vi "createChannel.vi"(8 "error in (no error)":errorcluster, 11 "SoundAO in":refnum<class "SoundAO.lvclass">) -> (0 "error out":errorcluster, 3 "SoundAO out":refnum<class "SoundAO.lvclass">)   [LabVIEW 2009, in "Hardware.lvlib" / "Channels.lvlib" / "SoundAO.lvclass"]
doc: "Abstract Method.\n\nCreates an analog output channel by reserving hardware resources needed by the output. This vi sets a name for the channel, and via its implementation classes (such as niDAQmxAO etc) reserves the physical channel on the output device."
uses:
  SoundAO.lvclass
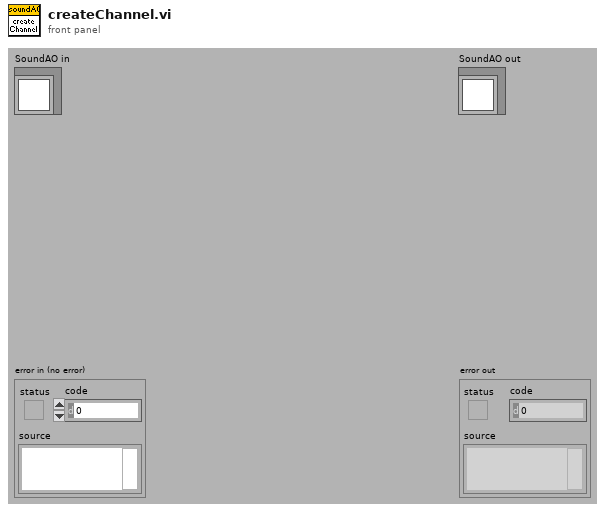
[diagram p1: front panel]
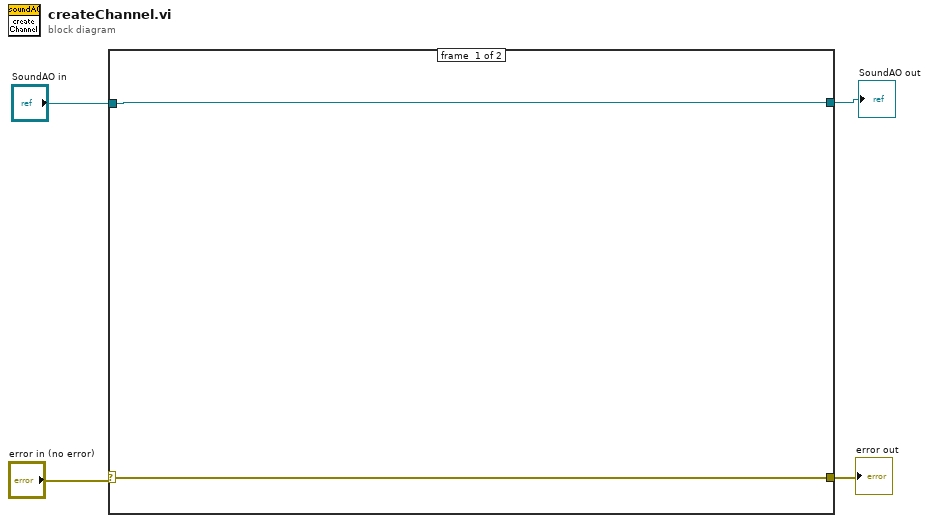
[diagram p0: block diagram]
diagram:
  n1 = case shown="No Error" "error in (no error)" {
    selector: "error in (no error)" -> [w6 w7]
    tunnel: [w6 w7] -> w3
    tunnel: "SoundAO in" -> [w5 w8]
    tunnel: [w5 w8] -> w1
    frame #0 {
    }
    frame #1 {
    }
  }
  "error out" <- w3
  "SoundAO out" <- w1
